vi "Test LV-WinSCP API.vi"() -> ()   [LabVIEW 2015]
doc: "LV-WinSCP API Tester."
uses:
  Classes/SessionOptions/SCP/SSHHostKeyPolicy.ctl
  Classes/Session/ListDirectory-Item.ctl
  Transfer Type.ctl
  Classes/FileTransfer/FileAndDestination.ctl
  Classes/FileTransfer/TransferExceptionDescription.ctl
  Classes/FileTransferOptions/TransferMode.ctl
  Classes/CommandExecution/ErrorDescription.ctl
  Classes/CommandExecution/Status.ctl
  <vilib>/Utility/error.llb/DialogType.ctl
  Classes/SessionOptions/SessionOptions.lvclass
  Classes/SessionOptions/SCP/SessionOptions-SCP.lvclass
  Classes/SessionOptions/FTP/SessionOptions-FTP.lvclass
  Classes/SessionOptions/SFTP/SessionOptions-SFTP.lvclass
  Classes/FileTransferOptions/FileTransferOptions.lvclass
  LV-WinSCP.lvlib
  Classes/Session/Session.lvclass
  Classes/FileTransfer/FileTransfer.lvclass
  Classes/CommandExecution/Command Execution.lvclass
panel:
  in  "Tab Control":T1(tab)
  in  "SessionType":enum32{"SCP", "FTP", "SFTP"}(tab)
  in  "SshHostKeyPolicy":T2=2 items=["Check", "GiveUpSecurityAndAcceptAny", "AcceptNew"]
  in  "Initialize Session":bool
  out "Connected?":bool
  in  "HostName":string="10.137.10.113"
  in  "UserName":string="admin"
  in  "PortNumber":i32=22
  in  "Password":string
  in  "Path":string
  in  "List Directory":bool
  out "Items Count":i32
  out "Items":T3[](array[typedef])
  in  "Get Items From Target":bool
  in  "Transfer Type":T4=enum."Folder"
  in  "wait for reply (T)":bool=TRUE
  out "File Transfered Successfully":T5[](array[typedef])
  out "Transfer Succeeded":bool
  out "Erroneous Transfers":T6[](array[typedef])
  in  "Local Path":path=path "C:/TransferSCP"
  in  "Path on Target":string="/etc"
  in  "Remove Items on Target":bool
  in  "PreserveTimestamp":bool
  in  "FileMask":string
  in  "TransferMode":T7
  in  "SpeedLimit(KB_s)":i32
  in  "Local Path Put":path=path "C:/Users/Public/Documents/National Instruments/CVI/samples/nisyscfg/BoardTemperatureMonitor" caption="Local Path"
  in  "Send Items To Target":bool
  in  "wait for reply (T) Put":bool=TRUE caption="wait for reply (T)"
  in  "Transfer Type Put":T4=enum."Folder" caption="Transfer Type"
  in  "Path on Target Put":string="/home/lvuser/Blip/" caption="Path on Target"
  in  "Remove Items on PC":bool
  in  "PreserveTimestamp Put":bool caption="PreserveTimestamp"
  in  "FileMask Put":string caption="FileMask"
  in  "TransferMode Put":T7 caption="TransferMode"
  in  "SpeedLimit(KB_s) Put":i32 caption="SpeedLimit(KB_s)"
  out "Transfer Succeeded Put":bool caption="Transfer Succeeded"
  out "Erroneous Transfers Put":T6[](array[typedef]) caption="Erroneous Transfers"
  out "File Transfered Successfully Put":T5[](array[typedef]) caption="File Transfered Successfully"
  in  "Execute Command On Target":bool
  in  "wait for reply - EC":bool=TRUE
  in  "Command":string
  out "EC - Status":T8
  out "EC - Errors":T9[](array[typedef])
  out "Sent Command":string
  out "Output":string
  in  "Close Session":bool
  in  "Show Diagram on Init":bool
  in  "Run as Singleton?":bool
  in  "Show Block Diagram":bool
  in  "Refresh Modules":bool
  out "Active Modules":string[](array[string])
  in  "Stop Module":bool
  in  "Select Module":i32(ring)=-1 caption="Select Module\nTo send Request to" items=["All"=-1, "0"=0]
  in  "Run New Module":bool
  in  "Hide Module Panel":bool
  in  "Show Module Panel":bool
  out "Status":string
  # "This VI tests the API for the Module."
  # "Nothing special to set here"
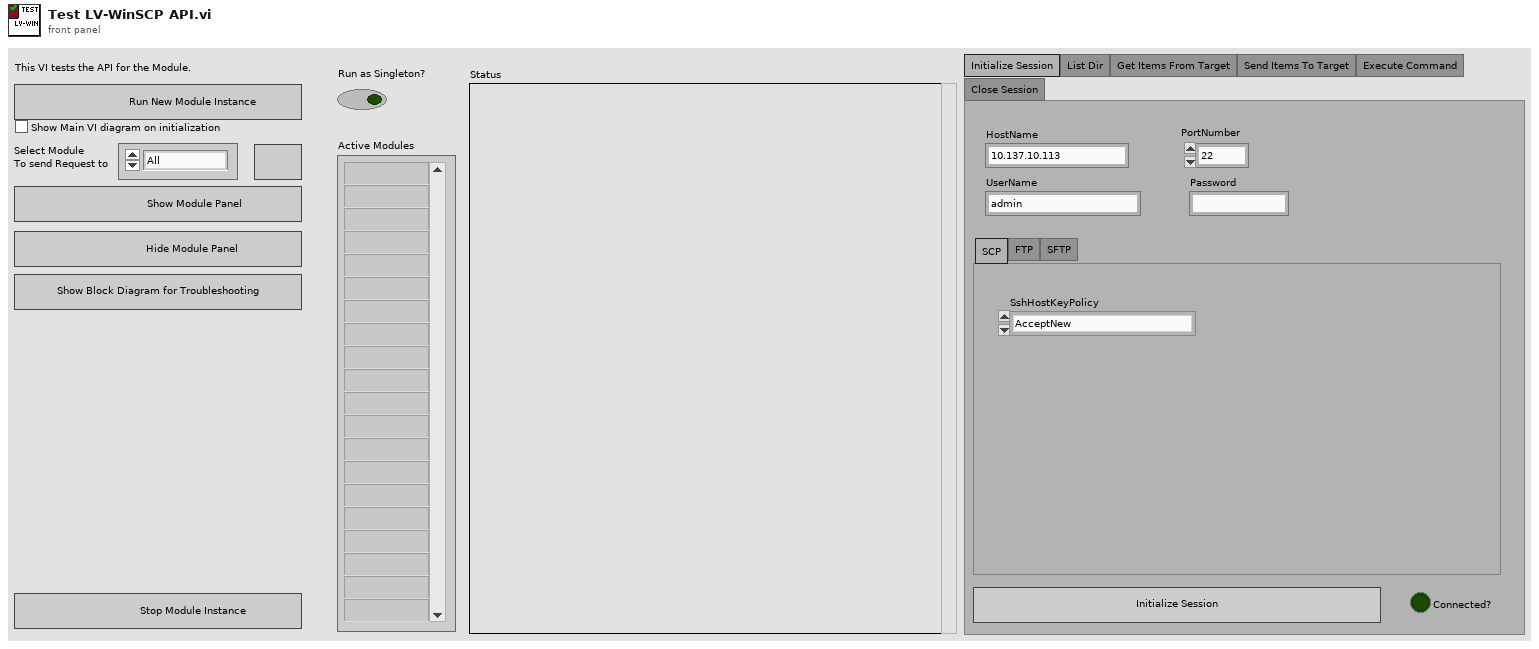
[diagram p1: front panel]
types:
  T1 = enum32{"Initialize Session", "List Dir", "Get Items From Target", "Send Items To Target", "Execute Command", "Close Session"}
  T2 = typedef "WinSCP.lvlib/SessionOptions-SCP.lvclass/SSHHostKeyPolicy.ctl" = i32
  T3 = typedef "WinSCP.lvlib/Session.lvclass/ListDirectory-Item.ctl" = cluster{"Name":string, "FullName":string, "FileType":u16, "Group":string, "Owner":string, "IsDirectory":bool, "IsParentDirectory":bool, "IsThisDirectory":bool, "LastWriteTime":timestamp, "Length":i64}
  T4 = typedef "LV-WinSCP.lvlib/Transfer Type.ctl" = enum16{"File", "Folder"}
  T5 = typedef "WinSCP.lvlib/FileTransfer.lvclass/FileAndDestination.ctl" = cluster{"FileName":string, "Destination":string}
  T6 = typedef "WinSCP.lvlib/FileTransfer.lvclass/TransferExceptionDescription.ctl" = cluster{"Message":string, "Source":string}
  T7 = typedef "WinSCP.lvlib/FileTransferOptions.lvclass/TransferMode.ctl" = enum16{"Binary", "Ascii", "Auto"}
  T8 = typedef "WinSCP.lvlib/Command Execution.lvclass/Status.ctl" = cluster{"IsSuccess":bool, "ErrorOutput":string, "ExitCode":i32}
  T9 = typedef "WinSCP.lvlib/Command Execution.lvclass/ErrorDescription.ctl" = cluster{"Message":string, "Source":string}
  T10 = typedef "LV-WinSCP.lvlib/Broadcast Events--cluster.ctl" = cluster{"Module Did Init":refnum<user-event>, "Status Updated":refnum<user-event>, "Error Reported":refnum<user-event>, "Module Did Stop":refnum<user-event>, "Update Module Execution Status":refnum<user-event>, "Transfer From Target Status":refnum<user-event>, "Command Execution Response":refnum<user-event>, "Transfer To Target Status":refnum<user-event>}
  T11 = typedef "DialogType.ctl" = u16
  T12 = typedef "LV-WinSCP.lvlib/Send Items To Target (Reply Payload)--cluster.ctl" = cluster{"Transfer Succeeded":bool, "File Transfered Successfully":T5[], "Erroneous Transfers":T6[], "error":errorcluster}
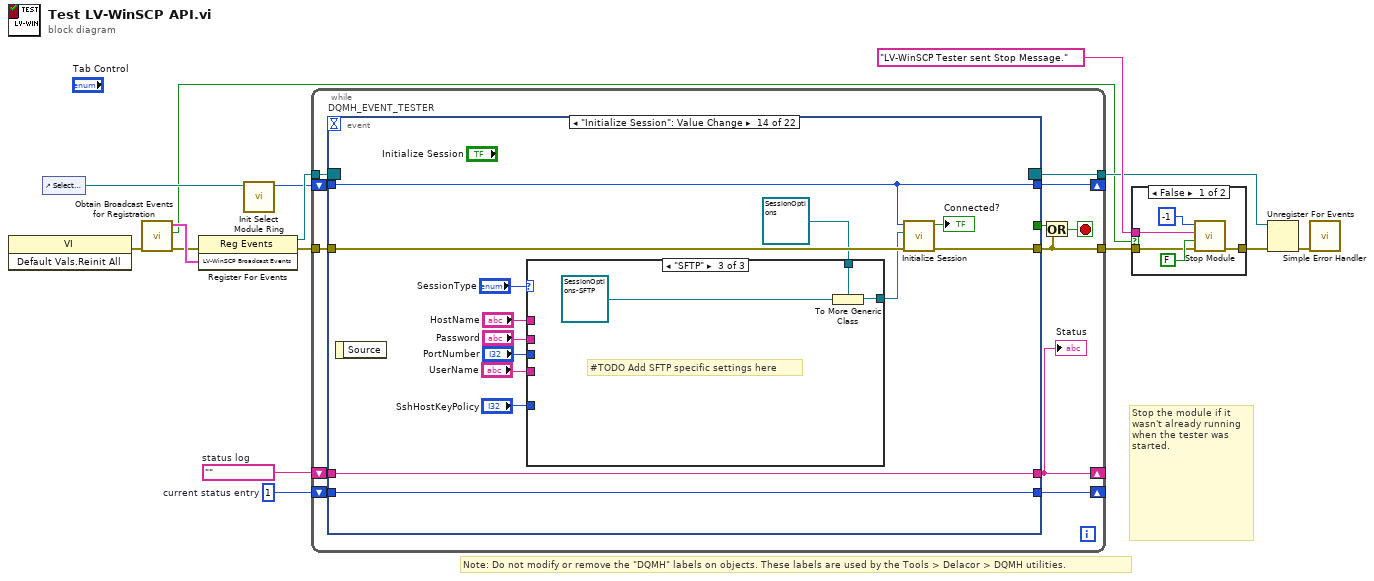
[diagram p0: block diagram]
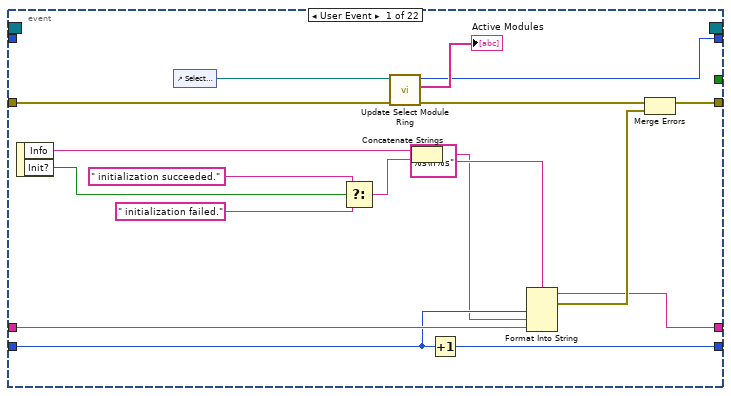
[diagram p3: hidden frame]
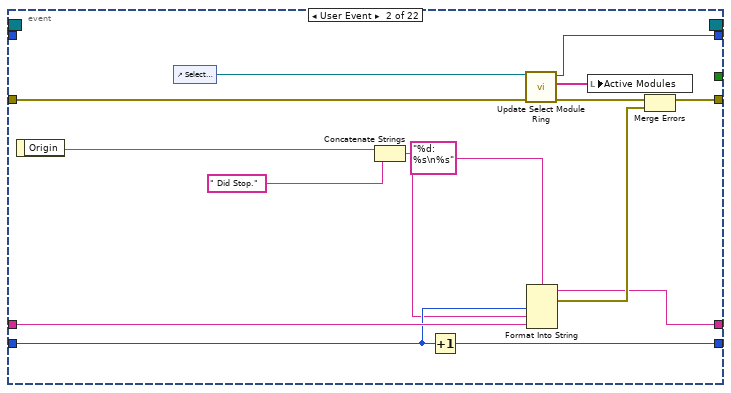
[diagram p4: hidden frame]
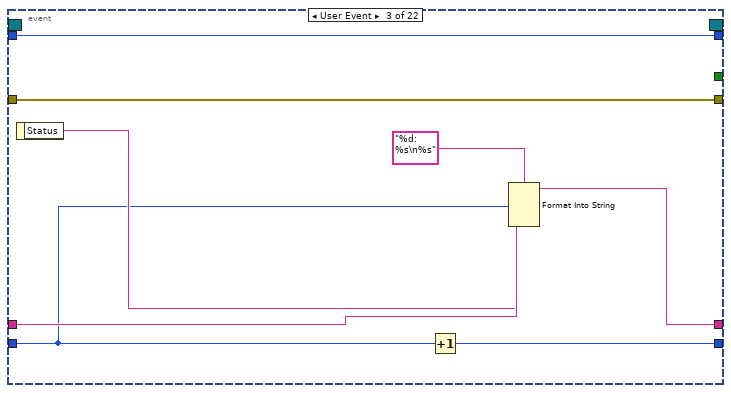
[diagram p5: hidden frame]
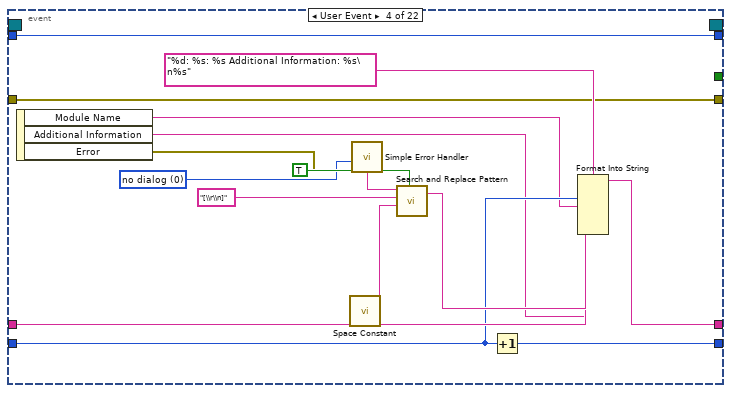
[diagram p6: hidden frame]
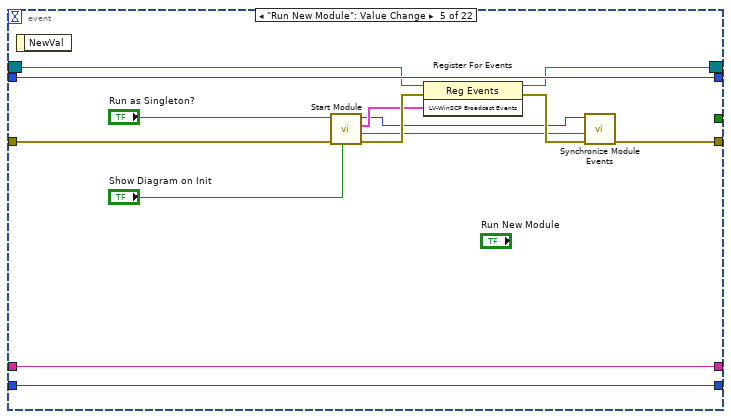
[diagram p7: hidden frame]
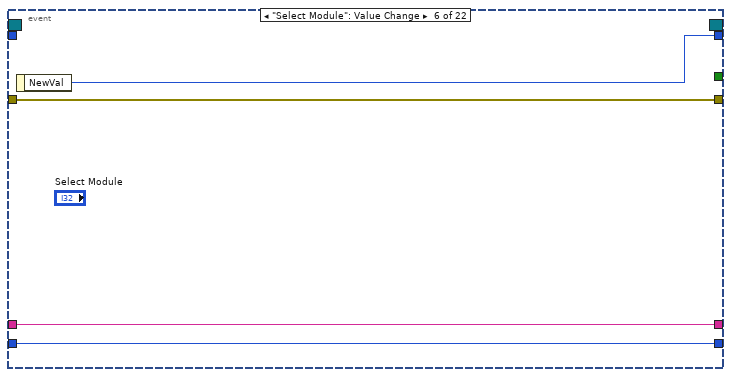
[diagram p8: hidden frame]
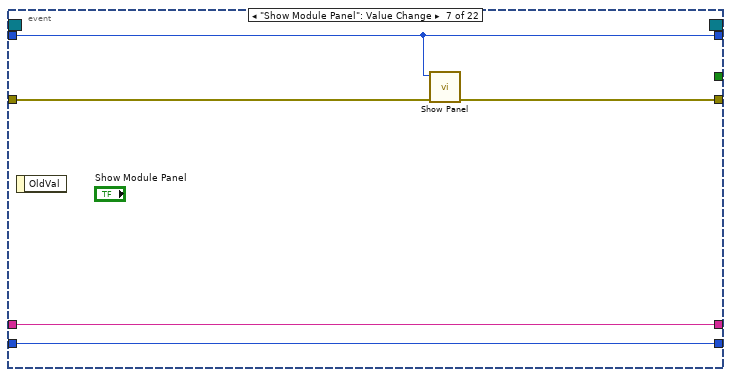
[diagram p9: hidden frame]
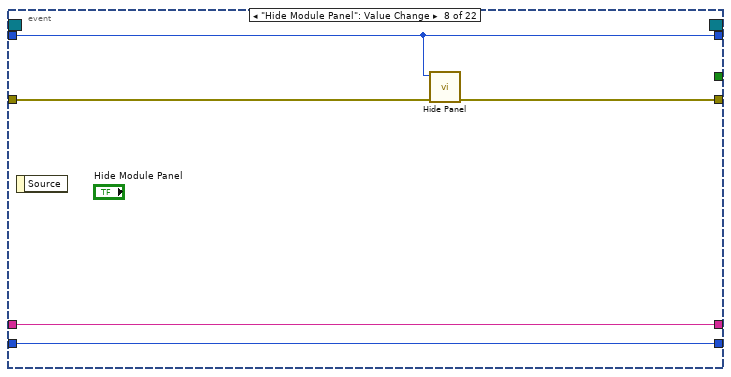
[diagram p10: hidden frame]
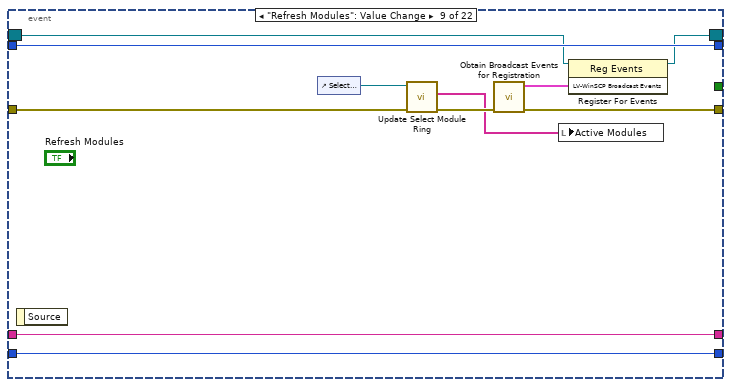
[diagram p11: hidden frame]
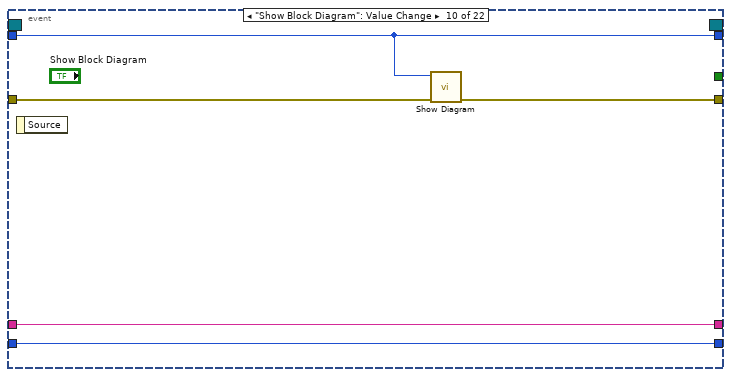
[diagram p12: hidden frame]
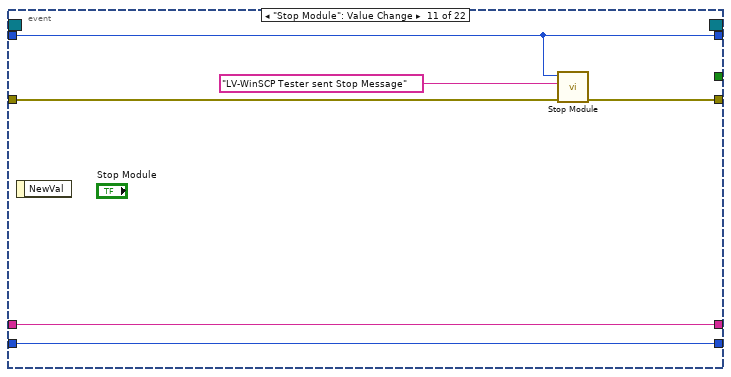
[diagram p13: hidden frame]
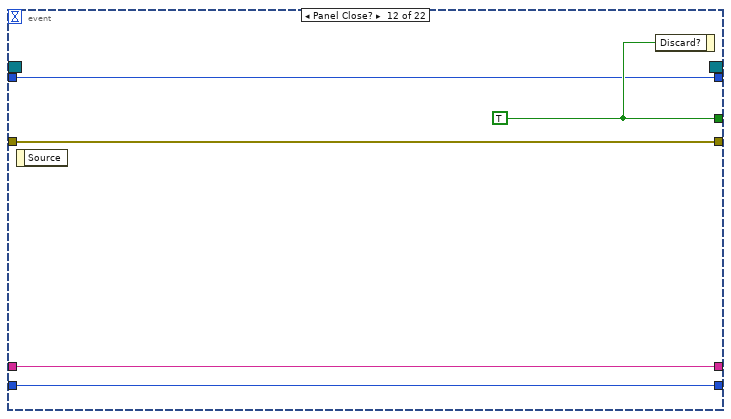
[diagram p14: hidden frame]
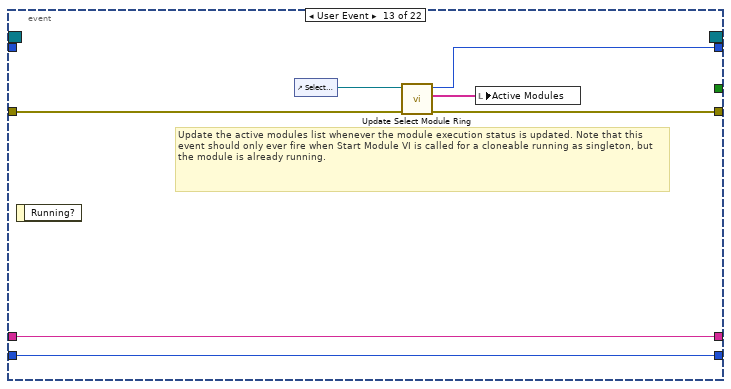
[diagram p15: hidden frame]
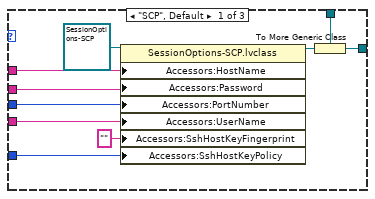
[diagram p16: hidden frame]
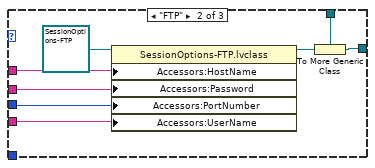
[diagram p17: hidden frame]
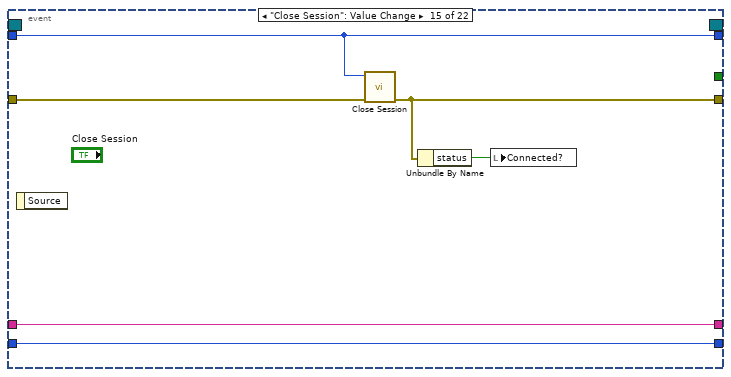
[diagram p18: hidden frame]
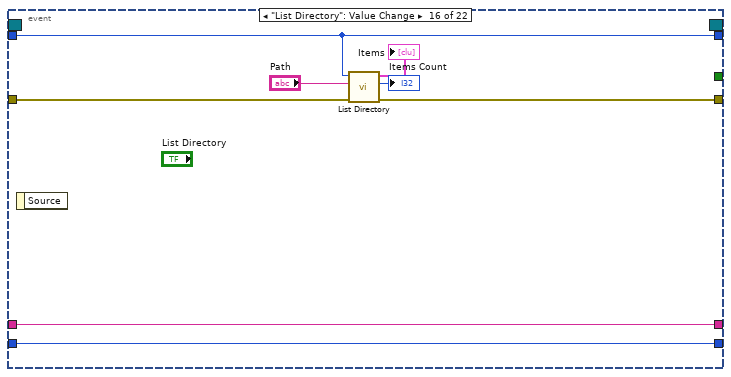
[diagram p19: hidden frame]
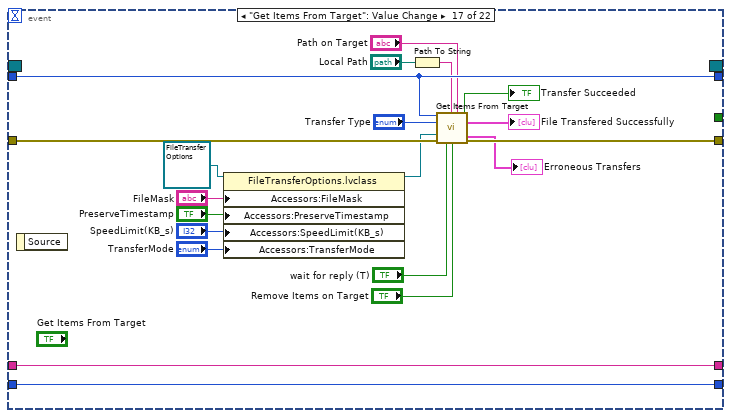
[diagram p20: hidden frame]
diagram:
  w12 = 1  # current status entry
  w13 = ""  # status log
  # "Stop the module if it wasn't already running when the tester was started."
  # "Note: Do not modify or remove the \"DQMH\" labels on objects. These labels are used by the Tools > Delacor > DQMH utilities."
  n1 = invoke class="VI" method="Default Vals.Reinit All"() -> (error out=w5:errorcluster)  [unwired: 3 in, 2 out]
  n2 = control-ref of="Select Module"() -> (w10:refnum<vi>)
  n3 = call "Obtain Broadcast Events for Registration.vi"("error in"=w5) -> ("error out"=w4:errorcluster, "Already running?"=w3:bool, "LV-WinSCP Broadcast Events"=w9:T10)  [unwired: 8 in]
  n4 = register-events(error in=w4, w9) -> (reference out=w15:refnum<event-registration>, error out=w8:errorcluster)  [unwired: 1 in]
  n5 = call "Init Select Module Ring.vi"("Select Module Ring Ref"=w10) -> ("Value for All Modules"=w11:i32)  [unwired: 8 in, 2 out]
  n6 = while {
    tunnel: w15 -> [w27]
    tunnel: [w16] -> w2
    tunnel: w8 -> [w25]
    shift-right: [w21] -> _
    shift-left: w13 -> [w23]
    shift-right: [w22] -> _
    shift-left: w12 -> [w24]
    shift-right: [w18] -> _
    shift-left: w11 -> [w19]
    tunnel: [w17] -> w6
    stop <- w20 stop-if-true
    n7 = event "DQMH_EVENT_TESTER" shown="[13] \"Initialize Session\": Value Change" {
      selector: w27 -> [_ _ _ _ w92 _ _ _ w118 _ _ _ _ _ _ _ _ _ _ _ _ _]
      dyn-events: [_ _ _ _ w91 _ _ _ w117 _ _ _ _ _ _ _ _ _ _ _ _ _] -> w17
      timeout: _ -> [_ _ _ _ _ _ _ _ _ _ _ _ _ _ _ _ _ _ _ _ _ _]
      tunnel: [_ _ _ _ _ _ _ _ _ _ _ w139 _ _ _ _ _ _ _ _ _ _] -> w26
      tunnel: [w35 w52 w68 w72 w90 w102 w106 w111 w114 w125 w130 w138 w142 w157 w183 w192 w212 w234 w242 w267 w290 w312] -> w16
      tunnel: w25 -> [w37 w54 w68 w72 w93 w102 w107 w112 w119 w128 w131 w138 w143 w160 w187 w195 w215 w234 w245 w267 w293 w312]
      tunnel: w24 -> [w42 w57 w61 w75 w95 w100 w104 w109 w122 w126 w133 w136 w145 w158 w185 w193 w213 w230 w243 w263 w291 w308]
      tunnel: w23 -> [w43 w58 w64 w76 w96 w101 w105 w110 w123 w127 w134 w137 w146 w159 w186 w194 w214 w232 w244 w265 w292 w310]
      tunnel: [w40 w55 w65 w74 w96 w101 w105 w110 w123 w127 w134 w137 w146 w159 w186 w194 w214 w231 w244 w264 w292 w309] -> w21
      tunnel: [w41 w56 w67 w73 w95 w100 w104 w109 w122 w126 w133 w136 w145 w158 w185 w193 w213 w229 w243 w262 w291 w307] -> w22
      tunnel: w19 -> [_ _ w62 w84 w94 _ w103 w108 w121 w124 w132 w135 _ w156 w184 w191 w211 w233 w241 w266 w289 w311]
      tunnel: [w32 w49 w62 w84 w94 w99 w103 w108 w121 w124 w132 w135 w141 w156 w184 w191 w211 w233 w241 w266 w289 w311] -> w18
      event User Event {
        n8 = event-data() -> ("Info"=w39:string, "Init?"=w29:bool)  [unwired: 1 in]
        n9 = control-ref of="Select Module"() -> (w34:refnum<vi>)
        n10 = Select(t=" initialization succeeded.", s=w29, f=" initialization failed.") -> (s? t:f=w28:string)
        n11 = call "Update Select Module Ring.vi"("error in (no error)"=w37, "Select Module Ring Ref"=w34) -> ("error out"=w36:errorcluster, "Active Modules (Array)"=→"Active Modules":string[], "New Module Ring Value"=w32:i32)  [unwired: 7 in]
        n12 = Concatenate Strings(w39, w28) -> (w38:string)
        n13 = Increment(x=w42) -> (x+1=w41:i32)
        n14 = Format Into String(format string="%d: %s\n%s", w42, w38, w43) -> (resulting string=w40:string, error out=w45:errorcluster)  [unwired: 2 in]
        n15 = Merge Errors(w36, w45) -> (w35:errorcluster)
      }
      event User Event {
        n16 = event-data() -> ("Origin"=w47:string)  [unwired: 1 in]
        n17 = control-ref of="Select Module"() -> (w51:refnum<vi>)
        n18 = Concatenate Strings(w47, " Did Stop.") -> (w46:string)
        n19 = Increment(x=w57) -> (x+1=w56:i32)
        n20 = call "Update Select Module Ring.vi"("error in (no error)"=w54, "Select Module Ring Ref"=w51) -> ("error out"=w53:errorcluster, "Active Modules (Array)"=w50:string[], "New Module Ring Value"=w49:i32)  [unwired: 7 in]
        n21 = Format Into String(format string="%d: %s\n%s", w57, w46, w58) -> (resulting string=w55:string, error out=w60:errorcluster)  [unwired: 2 in]
        n22 = local write "Active Modules"(w50) -> ()
        n23 = Merge Errors(w53, w60) -> (w52:errorcluster)
      }
      event User Event {
        n24 = event-data() -> ("Status"=w63:string)  [unwired: 1 in]
        n25 = Increment(x=w61) -> (x+1=w67:i32)
        n26 = Format Into String(format string="%d: %s\n%s", w61, w63, w64) -> (resulting string=w65:string)  [unwired: 2 in, 1 out]
      }
      event User Event {
        w77 = T11 0 items=["no dialog", "OK message", "continue or stop message", "OK message + warnings", "continue/stop + warnings"] ("type of dialog (OK msg:1)")
        n27 = event-data() -> ("Module Name"=w71:string, "Additional Information"=w70:string, "Error"=w69:errorcluster)  [unwired: 1 in]
        n28 = call <vilib>:"Space Constant.vi"() -> ("String"=w81:string)
        n29 = call <vilib>:"Simple Error Handler.vi"("type of dialog (OK msg:1)"=w77, "error in (no error)"=w69) -> ("message"=w78:string)  [unwired: 3 in, 4 out]
        n30 = call <vilib>:"Search and Replace Pattern.vi"("string"=w78, "regular expression (\"\")"="[\\r\\n]" ("regular expression (\"\")"), "replace string (\"\")"=w81, "replace all? (F)"=TRUE ("replace all CR/LF with spaces")) -> ("result string"=w79:string)  [unwired: 1 in, 1 out]
        n31 = Increment(x=w75) -> (x+1=w73:i32)
        n32 = Format Into String(format string="%d: %s: %s Additional Information: %s\n%s", w75, w71, w79, w70, w76) -> (resulting string=w74:string)  [unwired: 2 in, 1 out]
      }
      event "Run New Module": Value Change {
        n33 = event-data() -> ()  [unwired: 1 in, 1 out]
        n34 = call "Start Module.vi"("Show Main VI Diagram on Init (F)"="Show Diagram on Init", "error in"=w93, "Run as Singleton? (F)"="Run as Singleton?") -> ("error out"=w97:errorcluster, "Wait for Event Sync?"=w89:bool, "LV-WinSCP Broadcast Events"=w88:T10, "Module ID"=w85:i32)  [unwired: 5 in]
        n35 = register-events(reference=w92, error in=w97, w88) -> (reference out=w91:refnum<event-registration>, error out=w98:errorcluster)
        n36 = call "Synchronize Module Events.vi"("error in"=w98, "Wait for Event Sync?"=w89, "Module ID in"=w85) -> ("error out"=w90:errorcluster)  [unwired: 7 in, 1 out]
      }
      event "Select Module": Value Change {
        n37 = event-data() -> ("NewVal"=w99:i32)  [unwired: 1 in]
      }
      event "Show Module Panel": Value Change {
        n38 = event-data() -> ()  [unwired: 1 in, 1 out]
        n39 = call "Show Panel.vi"("error in (no error)"=w107, "Module ID"=w103) -> ("error out"=w106:errorcluster)  [unwired: 9 in]
      }
      event "Hide Module Panel": Value Change {
        n40 = event-data() -> ()  [unwired: 1 in, 1 out]
        n41 = call "Hide Panel.vi"("error in (no error)"=w112, "Module ID"=w108) -> ("error out"=w111:errorcluster)  [unwired: 9 in]
      }
      event "Refresh Modules": Value Change {
        n42 = event-data() -> ()  [unwired: 1 in, 1 out]
        n43 = control-ref of="Select Module"() -> (w120:refnum<vi>)
        n44 = call "Update Select Module Ring.vi"("error in (no error)"=w119, "Select Module Ring Ref"=w120) -> ("error out"=w115:errorcluster, "Active Modules (Array)"=w113:string[])  [unwired: 7 in, 1 out]
        n45 = call "Obtain Broadcast Events for Registration.vi"("error in"=w115) -> ("error out"=w114:errorcluster, "LV-WinSCP Broadcast Events"=w116:T10)  [unwired: 8 in, 1 out]
        n46 = local write "Active Modules"(w113) -> ()
        n47 = register-events(reference=w118, w116) -> (reference out=w117:refnum<event-registration>)  [unwired: 1 in, 1 out]
      }
      event "Show Block Diagram": Value Change {
        n48 = event-data() -> ()  [unwired: 1 in, 1 out]
        n49 = call "Show Diagram.vi"("error in (no error)"=w128, "Module ID"=w124) -> ("error out"=w125:errorcluster)  [unwired: 9 in]
      }
      event "Stop Module": Value Change {
        n50 = event-data() -> ()  [unwired: 1 in, 1 out]
        n51 = call "Stop Module.vi"("error in"=w131, "Origin"="LV-WinSCP Tester sent Stop Message", "Module ID"=w132) -> ("error out"=w130:errorcluster)  [unwired: 8 in]
      }
      event Panel Close? {
        w139 = TRUE ("Discard?")
        n52 = event-data() -> ()  [unwired: 1 in, 1 out]
        n53 = event-data("Discard?"=w139) -> ()  [unwired: 1 in, 1 out]
      }
      event User Event {
        # "Update the active modules list whenever the module execution status is updated. Note that this event should only ever fire when Start Module VI is called for a cloneable running as singleton, but the module is already running."
        n54 = event-data() -> ()  [unwired: 1 in, 1 out]
        n55 = control-ref of="Select Module"() -> (w144:refnum<vi>)
        n56 = call "Update Select Module Ring.vi"("error in (no error)"=w143, "Select Module Ring Ref"=w144) -> ("error out"=w142:errorcluster, "Active Modules (Array)"=w140:string[], "New Module Ring Value"=w141:i32)  [unwired: 7 in]
        n57 = local write "Active Modules"(w140) -> ()
      }
      event "Initialize Session": Value Change {
        n58 = event-data() -> ()  [unwired: 1 in, 1 out]
        n59 = case shown="\"SFTP\"" "SessionType" {
          tunnel: [w168 w175 w180] -> w153
          tunnel: refnum<class "SessionOptions.lvclass"> refnum ("SessionOptions.lvclass") -> [w167 w176 w181]
          tunnel: "HostName" -> [w165 w174 _]
          tunnel: "UserName" -> [w164 w171 _]
          tunnel: "Password" -> [w163 w173 _]
          tunnel: "PortNumber" -> [w162 w172 _]
          tunnel: "SshHostKeyPolicy" -> [w161 _ _]
          frame "SCP", Default {
            n60 = property class="SessionOptions-SCP.lvclass"(reference=refnum<class "SessionOptions-SCP.lvclass"> refnum ("SessionOptions-SCP.lvclass"), "Accessors:HostName"=w165, "Accessors:Password"=w163, "Accessors:PortNumber"=w162, "Accessors:UserName"=w164, "Accessors:SshHostKeyFingerprint"="" ("SshHostKeyFingerprint"), "Accessors:SshHostKeyPolicy"=w161) -> (reference out=w169:refnum<class "SessionOptions-SCP.lvclass">)  [unwired: 1 in, 1 out]
            n61 = To More Generic Class(target class=w167, reference=w169) -> (generic class reference=w168:refnum<class "SessionOptions.lvclass">)
          }
          frame "FTP" {
            n62 = property class="SessionOptions-FTP.lvclass"(reference=refnum<class "SessionOptions-FTP.lvclass"> refnum ("WinSCP.lvlib:SessionOptions-FTP.lvclass"), "Accessors:HostName"=w174, "Accessors:Password"=w173, "Accessors:PortNumber"=w172, "Accessors:UserName"=w171) -> (reference out=w177:refnum<class "SessionOptions-FTP.lvclass">)  [unwired: 1 in, 1 out]
            n63 = To More Generic Class(target class=w176, reference=w177) -> (generic class reference=w175:refnum<class "SessionOptions.lvclass">)
          }
          frame "SFTP" {
            # "#TODO Add SFTP specific settings here"
            n64 = To More Generic Class(target class=w181, reference=refnum<class "SessionOptions-SFTP.lvclass"> refnum ("WinSCP.lvlib:SessionOptions-SFTP.lvclass")) -> (generic class reference=w180:refnum<class "SessionOptions.lvclass">)
          }
        }
        n65 = call "Initialize Session.vi"("error in"=w160, "SessionOptions"=w153, "Module ID"=w156) -> ("error out"=w157:errorcluster, "Connected?"=→"Connected?":bool)  [unwired: 6 in, 1 out]
      }
      event "Close Session": Value Change {
        n66 = event-data() -> ()  [unwired: 1 in, 1 out]
        n67 = call "Close Session.vi"("error in"=w187, "Module ID"=w184) -> ("error out"=w183:errorcluster)  [unwired: 8 in, 1 out]
        n68 = Unbundle By Name(w183) -> ("status"=w182:bool)
        n69 = local write "Connected?"(w182) -> ()
      }
      event "List Directory": Value Change {
        n70 = event-data() -> ()  [unwired: 1 in, 1 out]
        n71 = call "List Directory.vi"("error in"=w195, "Path"="Path", "Module ID"=w191) -> ("error out"=w192:errorcluster, "Items Count"=→"Items Count":i32, "Items"=→"Items":T3[])  [unwired: 5 in, 1 out]
      }
      event "Get Items From Target": Value Change {
        n72 = event-data() -> ()  [unwired: 1 in, 1 out]
        n73 = property class="FileTransferOptions.lvclass"(reference=refnum<class "FileTransferOptions.lvclass"> refnum ("Transfer Options"), "Accessors:FileMask"="FileMask", "Accessors:PreserveTimestamp"="PreserveTimestamp", "Accessors:SpeedLimit(KB_s)"="SpeedLimit(KB_s)", "Accessors:TransferMode"="TransferMode") -> (reference out=w205:refnum<class "FileTransferOptions.lvclass">)  [unwired: 1 in, 1 out]
        n74 = Path To String(path="Local Path") -> (string=w198:string)
        n75 = call "Get Items From Target.vi"("Module ID"=w211, "Local Path"=w198, "Path on Target"="Path on Target", "Transfer Type"="Transfer Type", "Transfer Options"=w205, "error in"=w215, "wait for reply (T)"="wait for reply (T)", "Remove Items on Target"="Remove Items on Target") -> ("Transfer Succeeded"=→"Transfer Succeeded":bool, "File Transfered Successfully"=→"File Transfered Successfully":T5[], "Erroneous Transfers"=→"Erroneous Transfers":T6[], "error out"=w212:errorcluster)  [unwired: 3 in, 1 out]
      }
      event User Event {
        n76 = event-data() -> ("Transfer Succeeded"=w224:bool, "File Transfered Successfully"=w223:T5[], "Erroneous Transfers"=w222:T6[], "error"=w219:errorcluster)  [unwired: 1 in]
        n77 = Unbundle By Name(w219) -> ("code"=w218:i32, "source"=w217:string)
        n78 = Array Size(array=w223) -> (size(s)=w221:i32)
        n79 = Array Size(array=w222) -> (size(s)=w220:i32)
        n80 = Format Into String(format string="Transfer done : Success: %s ; Nb files transfered: %d ; Nb Erroneous Transfers: %d ; ERR: %d %s", w224, w221, w220, w218, w217) -> (resulting string=w216:string)  [unwired: 2 in, 1 out]
        n81 = Format Into String(format string="Response Received - %s", w216) -> (resulting string=w226:string)  [unwired: 2 in, 1 out]
        n82 = Increment(x=w230) -> (x+1=w229:i32)
        n83 = Format Into String(format string="%d: %s\n%s", w230, w226, w232) -> (resulting string=w231:string)  [unwired: 2 in, 1 out]
      }
      event "Execute Command On Target": Value Change {
        n84 = event-data() -> ()  [unwired: 1 in, 1 out]
        n85 = call "Execute Command On Target.vi"("wait for reply (T)"="wait for reply - EC", "error in"=w245, "Command"="Command", "Module ID"=w241) -> ("error out"=w242:errorcluster, "Errors"=→"EC - Errors":T9[], "Status"=→"EC - Status":T8, "Output"=→"Output":string, "Sent Command"=→"Sent Command":string)  [unwired: 2 in, 1 out]
      }
      event User Event {
        n86 = event-data() -> ("Sent Command"=w257:string, "Output"=w256:string, "Status"=w255:T8, "Errors"=w251:T9[])  [unwired: 1 in]
        n87 = Unbundle By Name(w255) -> ("IsSuccess"=w254:bool, "ErrorOutput"=w253:string, "ExitCode"=w252:i32)
        n88 = for {
          tunnel: w251 -> [w272] mode=indexing
          tunnel: [w268] -> w250 mode=indexing
          (unwired) "\r\n" ("End of Line Constant")
          n89 = Unbundle By Name(w272) -> ("Source"=w271:string, "Message"=w270:string)
          n90 = Concatenate Strings(w271, " ; " ("string"), w270) -> (w268:string)
        }
        n91 = Array To Spreadsheet String(delimiter (Tab)="\r\n" ("End of Line Constant"), array=w250, 3:"%s" ("format string")) -> (spreadsheet string=w247:string)
        n92 = Format Into String(format string="Cmd: %s\nOutput: \n%s\nSuccess: %s ; Err Output: %s ; ExitCode: %d ; Errors: \n%s", w257, w256, w254, w253, w252, w247) -> (resulting string=w246:string)  [unwired: 2 in, 1 out]
        n93 = Format Into String(format string="Response Received - %s", w246) -> (resulting string=w259:string)  [unwired: 2 in, 1 out]
        n94 = Increment(x=w263) -> (x+1=w262:i32)
        n95 = Format Into String(format string="%d: %s\n%s", w263, w259, w265) -> (resulting string=w264:string)  [unwired: 2 in, 1 out]
      }
      event "Send Items To Target": Value Change {
        n96 = event-data() -> ()  [unwired: 1 in, 1 out]
        n97 = property class="FileTransferOptions.lvclass"(reference=refnum<class "FileTransferOptions.lvclass"> refnum ("WinSCP.lvlib:FileTransferOptions.lvclass"), "Accessors:PreserveTimestamp"="PreserveTimestamp Put", "Accessors:SpeedLimit(KB_s)"="SpeedLimit(KB_s) Put", "Accessors:TransferMode"="TransferMode Put", "Accessors:FileMask"="FileMask Put") -> (reference out=w283:refnum<class "FileTransferOptions.lvclass">)  [unwired: 1 in, 1 out]
        n98 = Path To String(path="Local Path Put") -> (string=w281:string)
        n99 = call "Send Items To Target.vi"("Remove Items on PC"="Remove Items on PC", "Local Path"=w281, "wait for reply (T)"="wait for reply (T) Put", "Path on Target"="Path on Target Put", "error in"=w293, "TransferOptions"=w283, "Transfer Type"="Transfer Type Put", "Module ID"=w289) -> ("error out"=w290:errorcluster, "Reply Payload"=w276:T12)  [unwired: 1 in, 1 out]
        n100 = Unbundle(w276) -> ("Transfer Succeeded"=→"Transfer Succeeded Put":bool, "File Transfered Successfully"=→"File Transfered Successfully Put":T5[], "Erroneous Transfers"=→"Erroneous Transfers Put":T6[])  [unwired: 1 out]
      }
      event User Event {
        n101 = event-data() -> ("Transfer Succeeded"=w295:bool, "File Transfered Successfully"=w298:T5[], "Erroneous Transfers"=w297:T6[], "error"=w296:errorcluster)  [unwired: 1 in]
        n102 = Unbundle By Name(w296) -> ("code"=w300:i32, "source"=w299:string)
        n103 = Array Size(array=w298) -> (size(s)=w302:i32)
        n104 = Array Size(array=w297) -> (size(s)=w301:i32)
        n105 = Format Into String(format string="Transfer done : Success: %s ; Nb files transfered: %d ; Nb Erroneous Transfers: %d ; ERR: %d %s", w295, w302, w301, w300, w299) -> (resulting string=w294:string)  [unwired: 2 in, 1 out]
        n106 = Format Into String(format string="Response Received - %s", w294) -> (resulting string=w304:string)  [unwired: 2 in, 1 out]
        n107 = Increment(x=w308) -> (x+1=w307:i32)
        n108 = Format Into String(format string="%d: %s\n%s", w308, w304, w310) -> (resulting string=w309:string)  [unwired: 2 in, 1 out]
      }
    }
    "Status" <- w21
    n109 = Or(x=w26, y=w16) -> (x .or. y?=w20:bool)
  }
  n110 = case shown="False" w3 {
    tunnel: [w317 w318] -> w14
    tunnel: "LV-WinSCP Tester sent Stop Message." ("Origin") -> [w316 _]
    tunnel: w2 -> [w313 w318]
    frame False {
      n111 = call "Stop Module.vi"("error in"=w313, "Wait for Module to stop? (F)"=FALSE ("Wait for Module to stop?"), "Origin"=w316, "Module ID"=-1 ("Stop all")) -> ("error out"=w317:errorcluster)  [unwired: 7 in]
    }
    frame True {
    }
  }
  n112 = Unregister For Events(event registration refnum=w6, error in=w14) -> (error out=w1:errorcluster)
  n113 = call <vilib>:"Simple Error Handler.vi"("error in (no error)"=w1) -> ()  [unwired: 4 in, 5 out]
